vi "mac_mem_dot_32bit_mem_row1_22_outside.vi"(0 "StartIndex":u8, 1 "x_i":T2, 2 "Boolean":bool) -> (16 "ziyi_type":T1)   [LabVIEW 2017]
uses:
  x_qp_scalar.ctl
  ziyi_pipe_N22.ctl
  typeDefs/QP_mem_type.ctl
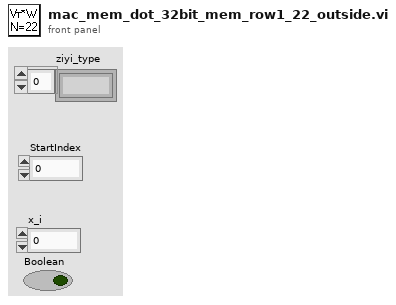
[diagram p1: front panel]
types:
  T1 = typedef "ziyi_pipe_N22.ctl" = T2[]
  T2 = typedef "x_qp_scalar.ctl" = fxp<+/-,32,6>
  T3 = typedef "QP_mem_type.ctl" = refnum<k21>
  T4 = typedef "xtype_scalar.ctl" = fxp<+/-,32,6>
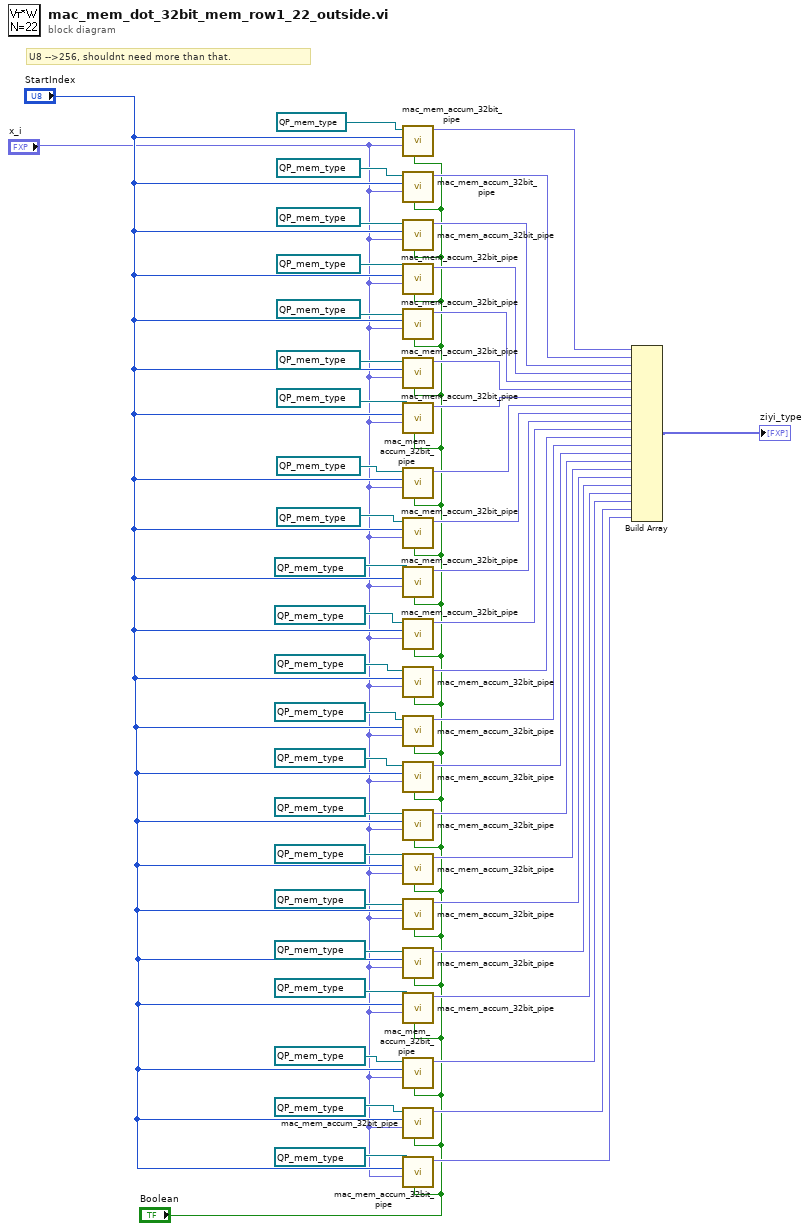
[diagram p0: block diagram]
diagram:
  # "U8 -->256, shouldnt need more than that."
  n1 = call "mac_mem_accum_32bit_pipe.vi"("sclr"="Boolean", "x_i"="x_i", "readIndex"="StartIndex", "QP-Memory"=T3 "Memory" ("Memory In")) -> ("s"=w47:T4)  [unwired: 7 in]
  n2 = call "mac_mem_accum_32bit_pipe.vi"("sclr"="Boolean", "x_i"="x_i", "readIndex"="StartIndex", "QP-Memory"=T3 "Memory 2" ("Memory In")) -> ("s"=w46:T4)  [unwired: 7 in]
  n3 = call "mac_mem_accum_32bit_pipe.vi"("sclr"="Boolean", "x_i"="x_i", "readIndex"="StartIndex", "QP-Memory"=T3 "Memory 3" ("Memory In")) -> ("s"=w45:T4)  [unwired: 7 in]
  n4 = call "mac_mem_accum_32bit_pipe.vi"("sclr"="Boolean", "x_i"="x_i", "readIndex"="StartIndex", "QP-Memory"=T3 "Memory 4" ("Memory In")) -> ("s"=w44:T4)  [unwired: 7 in]
  n5 = call "mac_mem_accum_32bit_pipe.vi"("sclr"="Boolean", "x_i"="x_i", "readIndex"="StartIndex", "QP-Memory"=T3 "Memory 5" ("Memory In")) -> ("s"=w43:T4)  [unwired: 7 in]
  n6 = call "mac_mem_accum_32bit_pipe.vi"("sclr"="Boolean", "x_i"="x_i", "readIndex"="StartIndex", "QP-Memory"=T3 "Memory 6" ("Memory In")) -> ("s"=w42:T4)  [unwired: 7 in]
  n7 = call "mac_mem_accum_32bit_pipe.vi"("sclr"="Boolean", "x_i"="x_i", "readIndex"="StartIndex", "QP-Memory"=T3 "Memory 7" ("Memory In")) -> ("s"=w41:T4)  [unwired: 7 in]
  n8 = call "mac_mem_accum_32bit_pipe.vi"("sclr"="Boolean", "x_i"="x_i", "readIndex"="StartIndex", "QP-Memory"=T3 "Memory 8" ("Memory In")) -> ("s"=w40:T4)  [unwired: 7 in]
  n9 = call "mac_mem_accum_32bit_pipe.vi"("sclr"="Boolean", "x_i"="x_i", "readIndex"="StartIndex", "QP-Memory"=T3 "Memory 9" ("Memory In")) -> ("s"=w39:T4)  [unwired: 7 in]
  n10 = call "mac_mem_accum_32bit_pipe.vi"("sclr"="Boolean", "x_i"="x_i", "readIndex"="StartIndex", "QP-Memory"=T3 "Memory 10" ("Memory In")) -> ("s"=w38:T4)  [unwired: 7 in]
  n11 = call "mac_mem_accum_32bit_pipe.vi"("sclr"="Boolean", "x_i"="x_i", "readIndex"="StartIndex", "QP-Memory"=T3 "Memory 11" ("Memory In")) -> ("s"=w37:T4)  [unwired: 7 in]
  n12 = call "mac_mem_accum_32bit_pipe.vi"("sclr"="Boolean", "x_i"="x_i", "readIndex"="StartIndex", "QP-Memory"=T3 "Memory 12" ("Memory In")) -> ("s"=w36:T4)  [unwired: 7 in]
  n13 = call "mac_mem_accum_32bit_pipe.vi"("sclr"="Boolean", "x_i"="x_i", "readIndex"="StartIndex", "QP-Memory"=T3 "Memory 13" ("Memory In")) -> ("s"=w12:T4)  [unwired: 7 in]
  n14 = call "mac_mem_accum_32bit_pipe.vi"("sclr"="Boolean", "x_i"="x_i", "readIndex"="StartIndex", "QP-Memory"=T3 "Memory 14" ("Memory In")) -> ("s"=w11:T4)  [unwired: 7 in]
  n15 = call "mac_mem_accum_32bit_pipe.vi"("sclr"="Boolean", "x_i"="x_i", "readIndex"="StartIndex", "QP-Memory"=T3 "Memory 15" ("Memory In")) -> ("s"=w10:T4)  [unwired: 7 in]
  n16 = call "mac_mem_accum_32bit_pipe.vi"("sclr"="Boolean", "x_i"="x_i", "readIndex"="StartIndex", "QP-Memory"=T3 "Memory 16" ("Memory In")) -> ("s"=w9:T4)  [unwired: 7 in]
  n17 = call "mac_mem_accum_32bit_pipe.vi"("sclr"="Boolean", "x_i"="x_i", "readIndex"="StartIndex", "QP-Memory"=T3 "Memory 17" ("Memory In")) -> ("s"=w8:T4)  [unwired: 7 in]
  n18 = call "mac_mem_accum_32bit_pipe.vi"("sclr"="Boolean", "x_i"="x_i", "readIndex"="StartIndex", "QP-Memory"=T3 "Memory 18" ("Memory In")) -> ("s"=w7:T4)  [unwired: 7 in]
  n19 = call "mac_mem_accum_32bit_pipe.vi"("sclr"="Boolean", "x_i"="x_i", "readIndex"="StartIndex", "QP-Memory"=T3 "Memory 19" ("Memory In")) -> ("s"=w6:T4)  [unwired: 7 in]
  n20 = call "mac_mem_accum_32bit_pipe.vi"("sclr"="Boolean", "x_i"="x_i", "readIndex"="StartIndex", "QP-Memory"=T3 "Memory 20" ("Memory In")) -> ("s"=w5:T4)  [unwired: 7 in]
  n21 = call "mac_mem_accum_32bit_pipe.vi"("sclr"="Boolean", "x_i"="x_i", "readIndex"="StartIndex", "QP-Memory"=T3 "Memory 21" ("Memory In")) -> ("s"=w4:T4)  [unwired: 7 in]
  n22 = call "mac_mem_accum_32bit_pipe.vi"("sclr"="Boolean", "x_i"="x_i", "readIndex"="StartIndex", "QP-Memory"=T3 "Memory 22" ("Memory In")) -> ("s"=w3:T4)  [unwired: 7 in]
  n23 = Build Array(w47, w46, w45, w44, w43, w42, w41, w40, w39, w38, w37, w36, w12, w11, w10, w9, w8, w7, w6, w5, w4, w3) -> (→"ziyi_type":T4[])
